vi "testSendCmdStatus.vi"(8 "error in (no error)":errorcluster) -> (0 "error out":errorcluster)   [LabVIEW 2018]
doc: "Test the sendCmdStatus.vi."
uses:
  src/TcpServer/TcpServer.lvclass
  src/TcpServerBase/typedef/tcpPacketTypeDef.ctl
  <vilib>/addons/_JKI Toolkits/Caraya/classes/Assert/Assert Equal Value_Variant.vi
  <vilib>/addons/_JKI Toolkits/Caraya/classes/Test/Test.lvclass
  <vilib>/addons/_JKI Toolkits/Caraya/classes/Assert/Assert.lvclass
  src/TcpServerCmd/TcpServerCmd.lvclass
  src/TcpServerBase/TcpServerBase.lvclass
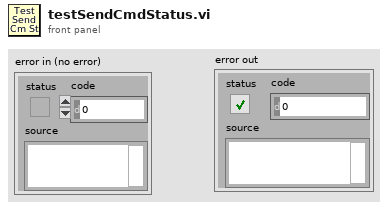
[diagram p1: front panel]
types:
  T1 = typedef "TcpServerBase.lvclass/tcpPacketTypeDef.ctl" = cluster{"packet":string, "firstPacket":bool, "firstConnection":bool}
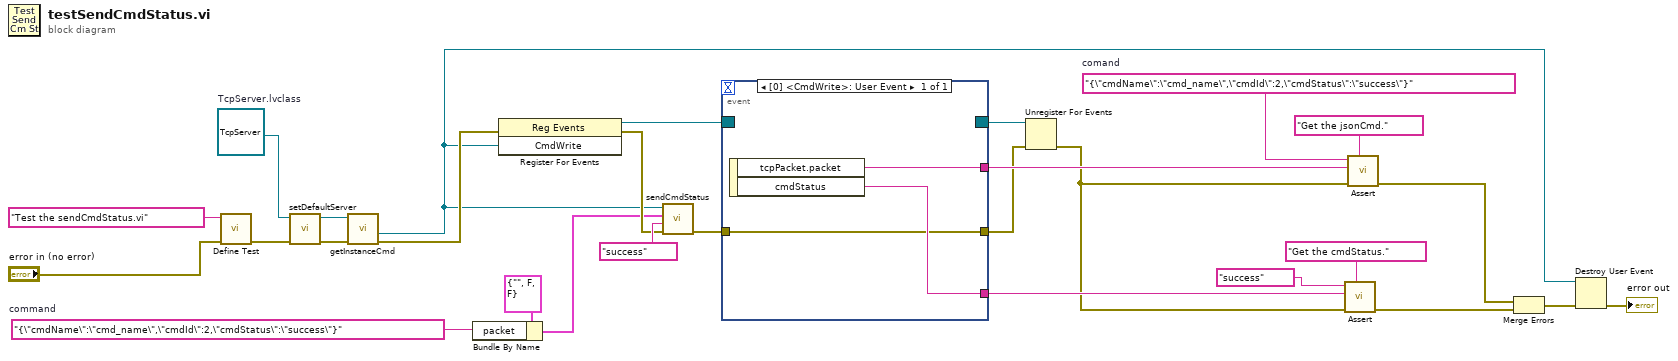
[diagram p0: block diagram]
diagram:
  w15 = "{\"cmdName\":\"cmd_name\",\"cmdId\":2,\"cmdStatus\":\"success\"}"  # comand
  w25 = refnum<class "TcpServer.lvclass"> refnum  # TcpServer.lvclass
  w3 = "{\"cmdName\":\"cmd_name\",\"cmdId\":2,\"cmdStatus\":\"success\"}"  # command
  n1 = call <vilib>:"Define Test.vi"("error in (no error)"="error in (no error)", "Label (VI Title)"="Test the sendCmdStatus.vi") -> ("error out"=w27:errorcluster)  [unwired: 9 in]
  n2 = call "setDefaultServer.vi"("error in (no error)"=w27, "TcpServer.lvclass"=w25) -> ("error out"=w5:errorcluster, "tcpServer out"=w6:refnum<class "TcpServer.lvclass">)  [unwired: 8 in]
  n3 = call "getInstanceCmd.vi"("error in (no error)"=w5, "tcpServer in"=w6) -> ("error out"=w7:errorcluster, "CmdWrite"=w1:refnum<user-event>)  [unwired: 6 in, 2 out]
  n4 = Bundle By Name(cluster=T1 {"packet"="", "firstPacket"=FALSE, "firstConnection"=FALSE} ("packetConnID"), "packet"=w3) -> (w2:T1)
  n5 = register-events(error in=w7, w1) -> (reference out=w23:refnum<event-registration>, error out=w22:errorcluster)  [unwired: 1 in]
  n6 = call "sendCmdStatus.vi"("error in (no error)"=w22, "cmdStatus"="success", "tcpPacket"=w2, "user event"=w1) -> ("error out"=w12:errorcluster)  [unwired: 7 in]
  n7 = event shown="[0] <CmdWrite>: User Event" {
    selector: w23 -> [_]
    dyn-events: [_] -> w11
    timeout: _ -> [_]
    tunnel: [w31] -> w19
    tunnel: [w30] -> w16
    tunnel: w12 -> [w29]
    tunnel: [w29] -> w10
    event User Event {
      n8 = event-data() -> ("tcpPacket.packet"=w30:string, "cmdStatus"=w31:string)  [unwired: 1 in]
    }
  }
  n9 = Unregister For Events(event registration refnum=w11, error in=w10) -> (error out=w9:errorcluster)
  n10 = call-poly <vilib>:"Assert.vi"("Label"="Get the cmdStatus.", "error in (no error)"=w9, "Y"=w19, "X"="success" ("cmdStatus")) -> ("error out"=w14:errorcluster)  [unwired: 7 in]
  n11 = call-poly <vilib>:"Assert.vi"("Label"="Get the jsonCmd.", "error in (no error)"=w9, "Y"=w16, "X"=w15) -> ("error out"=w13:errorcluster)  [unwired: 7 in]
  n12 = Merge Errors(w13, w14) -> (w21:errorcluster)
  n13 = Destroy User Event(user event=w1, error in=w21) -> (error out=→"error out":errorcluster)
